vi "DistancesAndTime.vi"(2 "Cluster XY Earth":cluster{dbl[], dbl[]}, 3 "Cluster XY Mars":cluster{dbl[], dbl[]}, 4 "Cluster XY Venus":cluster{dbl[], dbl[]}) -> (0 "time cluster":T1, 1 "distance cluster":T2)   [LabVIEW 2020]
doc: "Returns distance and time clusters containing information about distances between given input objects and time needed for information to flow between them."
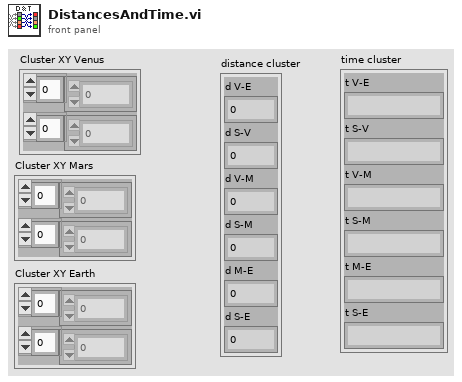
[diagram p1: front panel]
types:
  T1 = cluster{"t V-E":string, "t S-V":string, "t V-M":string, "t S-M":string, "t M-E":string, "t S-E":string}
  T2 = cluster{"d V-E":dbl, "d S-V":dbl, "d V-M":dbl, "d S-M":dbl, "d M-E":dbl, "d S-E":dbl}
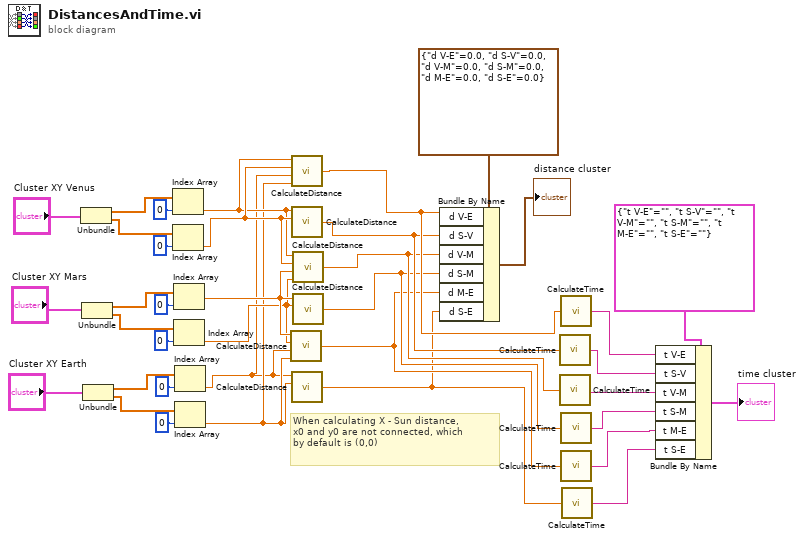
[diagram p0: block diagram]
diagram:
  # "When calculating X - Sun distance,\nx0 and y0 are not connected, which\nby default is (0,0)"
  n1 = Unbundle("Cluster XY Venus") -> (w36:dbl[], w34:dbl[])
  n2 = Unbundle("Cluster XY Mars") -> (w31:dbl[], w33:dbl[])
  n3 = Unbundle("Cluster XY Earth") -> (w28:dbl[], w26:dbl[])
  n4 = Index Array(array=w36, index=0) -> (element=w21:dbl)
  n5 = Index Array(array=w34, index=0) -> (element=w22:dbl)
  n6 = Index Array(array=w31, index=0) -> (element=w20:dbl)
  n7 = Index Array(array=w33, index=0) -> (element=w19:dbl)
  n8 = Index Array(array=w28, index=0) -> (element=w17:dbl)
  n9 = Index Array(array=w26, index=0) -> (element=w18:dbl)
  n10 = call "CalculateDistance.vi"("y0"=w18, "x0"=w17, "y"=w19, "x"=w20) -> ("distance"=w10:dbl)
  n11 = call "CalculateDistance.vi"("y0"=w18, "x0"=w17, "y"=w22, "x"=w21) -> ("distance"=w14:dbl)
  n12 = call "CalculateDistance.vi"("y"=w22, "x"=w21) -> ("distance"=w13:dbl)  [unwired: 2 in]
  n13 = call "CalculateDistance.vi"("y"=w18, "x"=w17) -> ("distance"=w9:dbl)  [unwired: 2 in]
  n14 = call "CalculateDistance.vi"("y0"=w19, "x0"=w20, "y"=w22, "x"=w21) -> ("distance"=w12:dbl)
  n15 = call "CalculateDistance.vi"("y"=w19, "x"=w20) -> ("distance"=w11:dbl)  [unwired: 2 in]
  n16 = Bundle By Name(cluster=T2 {"d V-E"=0.0, "d S-V"=0.0, "d V-M"=0.0, "d S-M"=0.0, "d M-E"=0.0, "d S-E"=0.0}, "d V-E"=w14, "d S-V"=w13, "d V-M"=w12, "d S-M"=w11, "d M-E"=w10, "d S-E"=w9) -> (→"distance cluster":T2)
  n17 = call "CalculateTime.vi"("distance"=w13) -> ("time min:s:ms"=w6:string)
  n18 = call "CalculateTime.vi"("distance"=w12) -> ("time min:s:ms"=w5:string)
  n19 = call "CalculateTime.vi"("distance"=w14) -> ("time min:s:ms"=w7:string)
  n20 = call "CalculateTime.vi"("distance"=w11) -> ("time min:s:ms"=w4:string)
  n21 = call "CalculateTime.vi"("distance"=w10) -> ("time min:s:ms"=w3:string)
  n22 = call "CalculateTime.vi"("distance"=w9) -> ("time min:s:ms"=w2:string)
  n23 = Bundle By Name(cluster=T1 {"t V-E"="", "t S-V"="", "t V-M"="", "t S-M"="", "t M-E"="", "t S-E"=""}, "t V-E"=w7, "t S-V"=w6, "t V-M"=w5, "t S-M"=w4, "t M-E"=w3, "t S-E"=w2) -> (→"time cluster":T1)
